vi "RSZVB File Manager.vi"(7 "Destination":string, 8 "error in (no error)":errorcluster {"code" format="%.0x"}, 9 "Source (D:\\user\\data)":string="D:\\user\\data", 10 "Operation to be Performed (0: Change Drive)":i32(ring) items=["Change Drive", "Change Current Directory", "Create Directory", "Delete Directory", "Copy File", "Move File", "Delete File", "Select default directory"], 11 "VISA session":refnum<visa-resource-name>) -> (0 "error out":errorcluster {"code" format="%.0x"}, 3 "dup VISA session":refnum<visa-resource-name>)   [LabVIEW 2011]
doc: "This VI provides operations which allows to do basic file operations on the storage media of the instrument. It consists from the following operations:\n\n Change Drive\n Change Current Directory\n Create Directory\n Delete Directory\n Copy File\n Move File\n Delete File\n\nRemote-control command(s):\nMMEMory:MSIS '<device>'\nMMEMory:CDIRectory '<directory_name>'\nMMEMory:MDIRectory '<directory_name>'\nMMEMory:RDIRectory '<directory_name>'\nMMEMory:COPY '<file_source>','<file_destination>'\nMMEMory:MOVE '<file_source>','<file_destination>'\nMMEMory:DELete '<file_name>'"
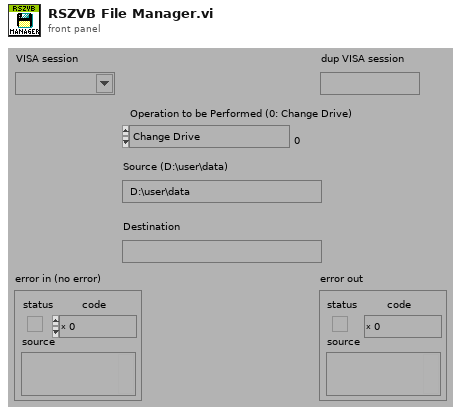
[diagram p1: front panel]
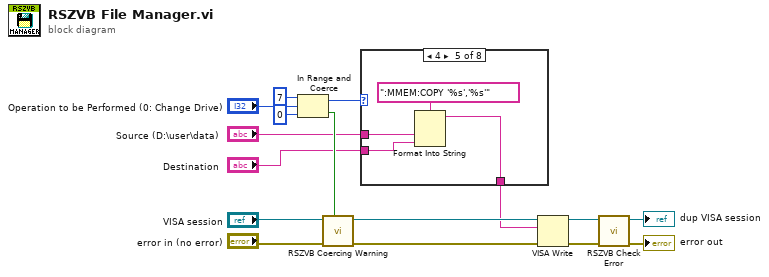
[diagram p0: block diagram]
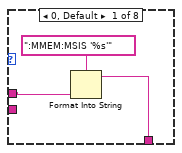
[diagram p2: hidden frame]
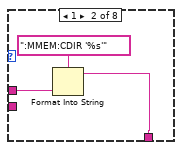
[diagram p3: hidden frame]
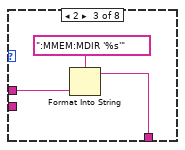
[diagram p4: hidden frame]
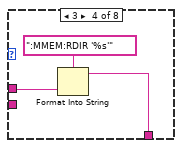
[diagram p5: hidden frame]
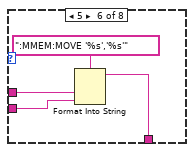
[diagram p6: hidden frame]
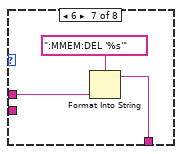
[diagram p7: hidden frame]
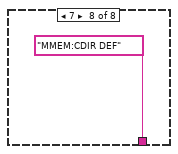
[diagram p8: hidden frame]
diagram:
  n1 = In Range and Coerce(upper limit=7, x="Operation to be Performed (0: Change Drive)", lower limit=0) -> (coerced(x)=w14:i32, In Range?=w5:bool)
  n2 = call "RSZVB Coercing Warning.vi"("In Range?"=w5, "error in (no error)"="error in (no error)", "VISA session"="VISA session") -> ("error out"=w9:errorcluster, "dup VISA session"=w8:refnum<visa-resource-name>)  [unwired: 7 in]
  n3 = case shown="4" w14 {
    tunnel: [w18 w21 w23 w26 w29 w33 w37 "MMEM:CDIR DEF"] -> w2
    tunnel: "Source (D:\\user\\data)" -> [w17 w20 w24 w27 w31 w35 w38 _]
    tunnel: "Destination" -> [_ _ _ _ w30 w34 _ _]
    frame 0, Default {
      n4 = Format Into String(format string=":MMEM:MSIS '%s'", w17) -> (resulting string=w18:string)  [unwired: 2 in, 1 out]
    }
    frame 1 {
      n5 = Format Into String(format string=":MMEM:CDIR '%s'", w20) -> (resulting string=w21:string)  [unwired: 2 in, 1 out]
    }
    frame 2 {
      n6 = Format Into String(format string=":MMEM:MDIR '%s'", w24) -> (resulting string=w23:string)  [unwired: 2 in, 1 out]
    }
    frame 3 {
      n7 = Format Into String(format string=":MMEM:RDIR '%s'", w27) -> (resulting string=w26:string)  [unwired: 2 in, 1 out]
    }
    frame 4 {
      n8 = Format Into String(format string=":MMEM:COPY '%s','%s'", w31, w30) -> (resulting string=w29:string)  [unwired: 2 in, 1 out]
    }
    frame 5 {
      n9 = Format Into String(format string=":MMEM:MOVE '%s','%s'", w35, w34) -> (resulting string=w33:string)  [unwired: 2 in, 1 out]
    }
    frame 6 {
      n10 = Format Into String(format string=":MMEM:DEL '%s'", w38) -> (resulting string=w37:string)  [unwired: 2 in, 1 out]
    }
    frame 7 {
    }
  }
  n11 = VISA Write(VISA resource name=w8, write buffer=w2, error in (no error)=w9) -> (VISA resource name out=w11:refnum<visa-resource-name>, error out=w10:errorcluster)  [unwired: 1 out]
  n12 = call "RSZVB Check Error.vi"("error in (no error)"=w10, "VISA session"=w11) -> ("error out"=→"error out":errorcluster, "dup VISA session"=→"dup VISA session":refnum<visa-resource-name>)  [unwired: 8 in]
